vi "Functional Imaging-Update UI element limits.vi"(8 "error in (no error)":errorcluster) -> (0 "error out":errorcluster)   [LabVIEW 2017]
uses:
  Experiment header interface/Typedefs/Header file interface module functions enum.ctl
  Typedefs/Get-Set-Clear Control.ctl
  Global variables/gl_Functional Imaging-Global variables.vi
panel:
  out "Experiment data folder path":path
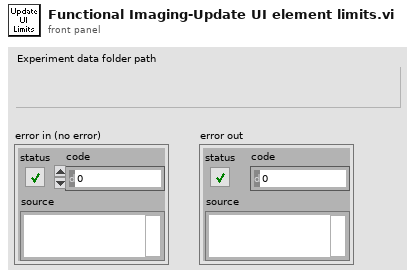
[diagram p1: front panel]
types:
  T1 = typedef "Header file interface module functions enum.ctl" = enum16{"Load experiment header file", "Save experiment header file", "Clear stored values", "Read stored values", "Update specific value in memory", "Update values in memory"}
  T2 = typedef "Functional Imging UI Refs.ctl" = cluster{"Menu ref":refnum<k9>, "Image control":refnum<vi>, "VI ref":refnum<vi>, "XGrapher":refnum<vi>, "Smoothing":refnum<vi>, "POI Averaging":refnum<vi>, "Normalize":refnum<vi>, "POI data points in each trial":refnum<vi>, "Channel":refnum<vi>, "Experiment data folder path":refnum<vi>, "[ROI vis]":refnum<vi>, "[Groups] visbl":T3, "Group Name":refnum<vi>, "POI index":refnum<vi>, "Trial No.":refnum<vi>, "Intensity Zoom":refnum<vi>, "Trial Cursor Enabled":refnum<vi>, "Number of Trials (ind 1)":refnum<vi>, "Number of Trials (ind 2)":refnum<vi>, "MiniScans Available":refnum<vi>, "POI Available":refnum<vi>, "Defer graph updates":refnum<vi>, "Waveform selector":refnum<vi>, "#of selected POI":refnum<vi>, "#of selected MiniScans":refnum<vi>, "#of selected groups":refnum<vi>, "Max Z-Projection":refnum<vi>, "Z-Plane Selector":refnum<vi>, "Index of miniscan point to visualise":refnum<vi>, "ROI vis. mode":refnum<vi>, "Total # of points":refnum<vi>, "Index of group clicked on":refnum<vi>, "Pane 1":refnum<vi>, "Pane 2":refnum<vi>, "Pane 3":refnum<vi>, "Pane 4":refnum<vi>, "Pane 5":refnum<vi>, "Pane 6":refnum<vi>, "Deselect all ROI":refnum<vi>, "Deselect all groups":refnum<vi>}
  T3 = typedef "Groups array referecne.ctl" = refnum<vi>
  T4 = typedef "Header parameters cluster-ALL.ctl" = cluster{"LOGIN":T5, "GLOBAL PARAMETERS":T6, "IMAGING MODES":T8, "TIME SERIES":T9, "MOTOR Z-STACK ":T11, "AOL Z-STACK":T12, "FUNCTIONAL IMAGING":T13, "MOVEMENT CORRECTION":T14, "CALIBRATION":T16, "STATISTICS":T17, "BIOLOGY INFORMATION":T18}
  T5 = typedef "Header params -Login.ctl" = cluster{"User":string, "Profile":string, "Software Version":string, "Experiment Date Time":timestamp}
  T6 = typedef "Header params-Global Parameters.ctl" = cluster{"MicroscopeID":string, "Microscope Type":string, "Objective":string, "Field of View (um)":dbl, "Fill time (us)":dbl, "Experiment Type":T7, "Stimuli Trigger":bool, "Speed Logging":bool}
  T7 = typedef "Experiment Type.ctl" = enum16{"In vivo", "In vitro", "Testing", "Calibration", "Other"}
  T8 = typedef "Header params-Imaging Modes.ctl" = cluster{"Time Series":bool, "Motor Zstack":bool, "AOL Zstack":bool, "Functional Imaging":bool}
  T9 = typedef "Header params-Time Series.ctl" = cluster{"Basic Image meta data":T10, "AOL z":dbl}
  T10 = typedef "Header params-Basic image meta data.ctl" = cluster{"Wavelength (nm)":dbl, "# averaged frames":dbl, "laser power (%)":dbl, "Pockels":dbl, "pixel dwell time (us)":dbl, "fill time (us)":dbl, "pmt 1":dbl, "pmt 2":dbl, "back apperture":dbl, "zoom":dbl, "field of view":dbl, "frame size":dbl, "AOL x centre":dbl, "AOL y centre":dbl, "Stage x position":dbl, "Stage y position":dbl, "Stage z position":dbl}
  T11 = typedef "Header params-Motor Z-stack.ctl" = cluster{"Hdr Basic Image meta data":T10, "Z Start":dbl, "Z Stop":dbl, "No of Planes":dbl}
  T12 = typedef "Header params-AOL Z-stack.ctl" = cluster{"Hdr Basic Image meta data":T10, "Z Start":dbl, "Z Stop":dbl, "No of Planes":dbl}
  T13 = typedef "Header params-Functional Imaging.ctl" = cluster{"Functional Mode":enum16{"Point", "Line", "Patch", "Plane", "Volume"}, "Pockels Modulation":bool, "Number of pois":dbl, "Number of miniscans":dbl, "Number of cycles":dbl, "Number of trials":dbl, "Miniscan dwell time per pixel (us)":dbl, "poi dwell time":dbl, "Rectangle ROI length":dbl, "Rectangle ROI height":dbl, "AOL mode":dbl, "Plane mode":dbl, "video length (sec)":dbl, "Frame rate (fps)":dbl, "Stimuli Timing (usec)":dbl, "Acquisition Length":dbl, "Basic Image meta data":T10, "Z Start (um)":dbl, "Z Stop (um)":dbl}
  T14 = typedef "Header params-Movement correction.ctl" = cluster{"Movement Correction":bool, "Axial Reference":bool, "Reference Size":dbl, "Reference Source":T15, "Reference dwell time (us)":dbl, "Number of Z lines":dbl, "Size of Z pixels":dbl, "Axial Pixels":dbl, "Reference Zoom":dbl, "Reference Average":dbl, "Proportional Scale":dbl, "Integral Scale":dbl, "Proportional Scale Z":dbl, "Integral Scale Z":dbl, "Scan Interval":dbl, "Ref Plot Refresh Rate":dbl}
  T15 = typedef "Reference source.ctl" = enum16{"Green channel", "Red channel"}
  T16 = typedef "Header params-Calibration Setup.ctl" = cluster{"Pockels Calibration File":path, "Calibration_ini file":path, "Setup_ini file":path}
  T17 = typedef "Header params-statistics.ctl" = cluster{"Z-stack duration (sec)":dbl, "Number of acquired data-points":dbl, "Acquisition time (ms)":dbl, "Number of acquired frames":dbl}
  T18 = typedef "Biology Information.ctl" = cluster{"Animal Code or Name":string, "Animal DoB":string, "Animal Age":string, "Animal Sex":string, "Animal Weight":string, "Date of Injection":string, "Date of Implant":string, "Site of Injection":string, "Animal Ear Notch":string, "AAV constructs":string, "Genetic background":string, "Optical reporter":string, "Region of brain imaged":string, "Other \ncomments":string}
  T19 = typedef "Get-Set-Clear Control.ctl" = enum16{"Get", "Set", "Clear"}
  T20 = typedef "Fixed strings.ctl" = cluster{"ROI file name":string, "Normalised ROI file name":string, "Zplane Pockels values file name":string, "Functional data folder name":string, "Experiment Header file name":string, "Z-stack images folder name":string, "Groups setup rel. path":string, "Groups text file rel. path":string, "TDMS files folder name (F.img)":string, "TDMS files folder name (V.acq)":string, "TDMS files folder name (Pl.acq)":string, "Cycle rel times sequence file":string, "Dynamically called VIs folder name":string, "Time Series folder base name":string}
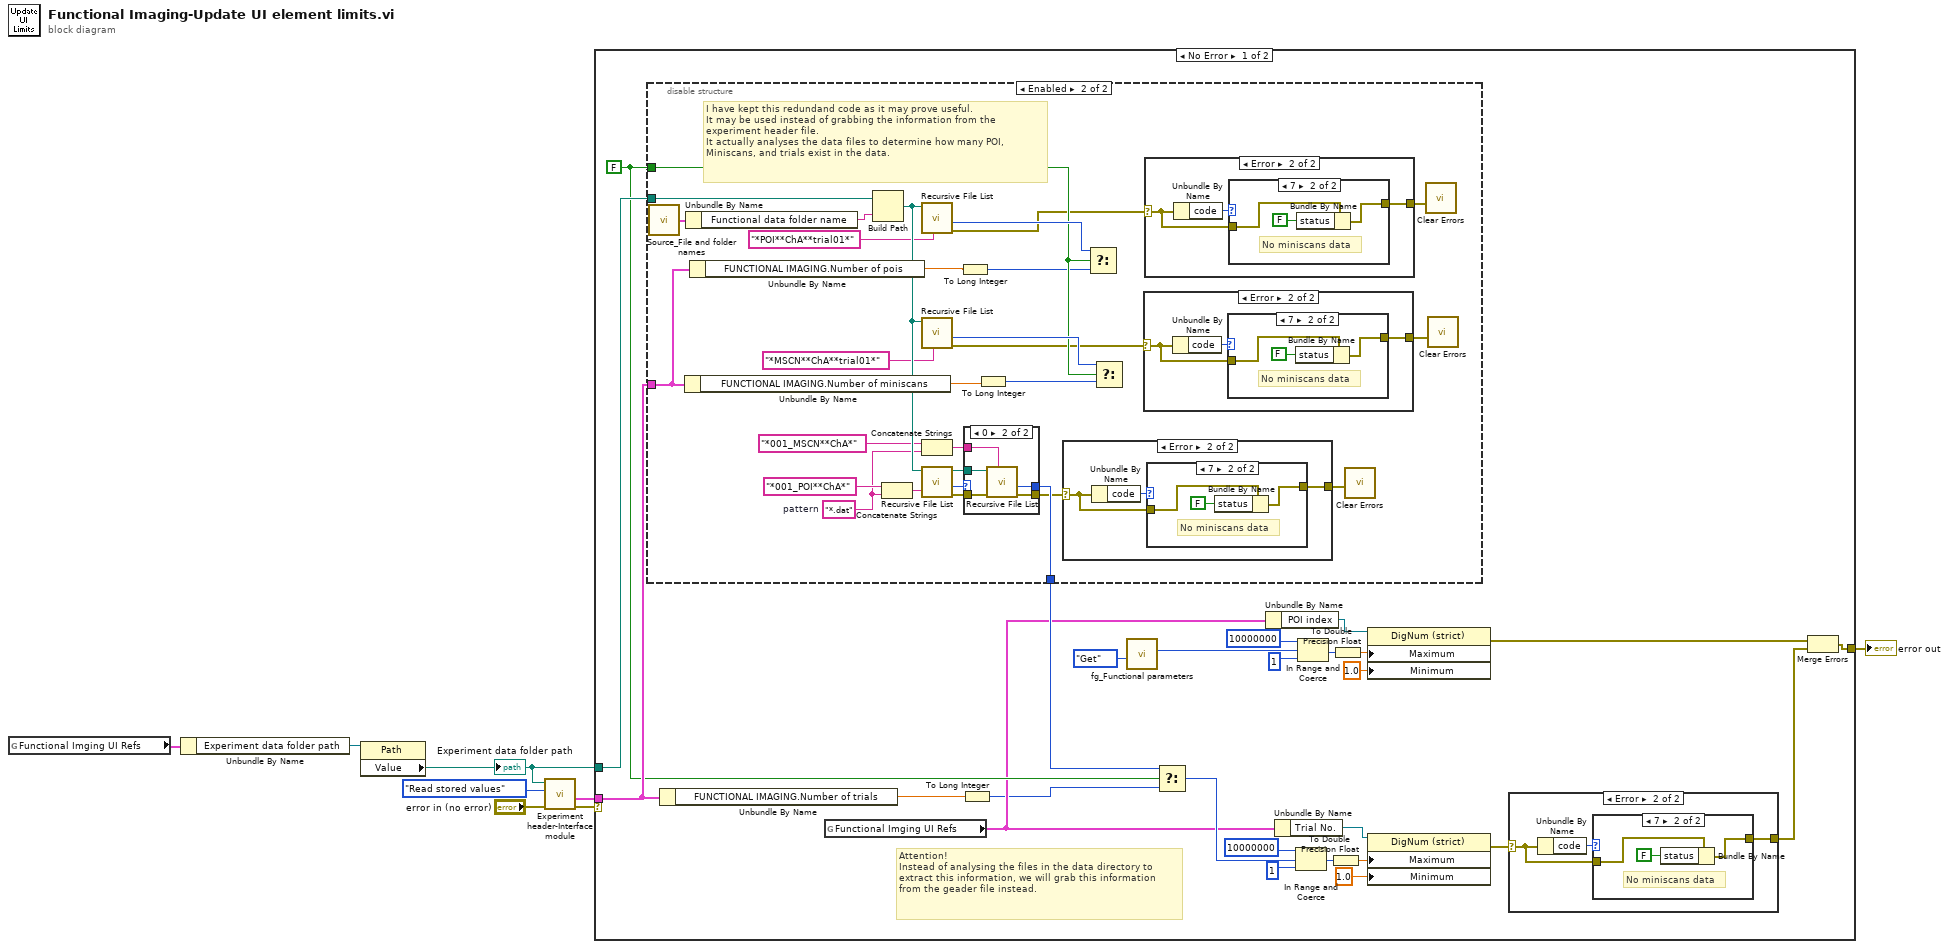
[diagram p0: block diagram]
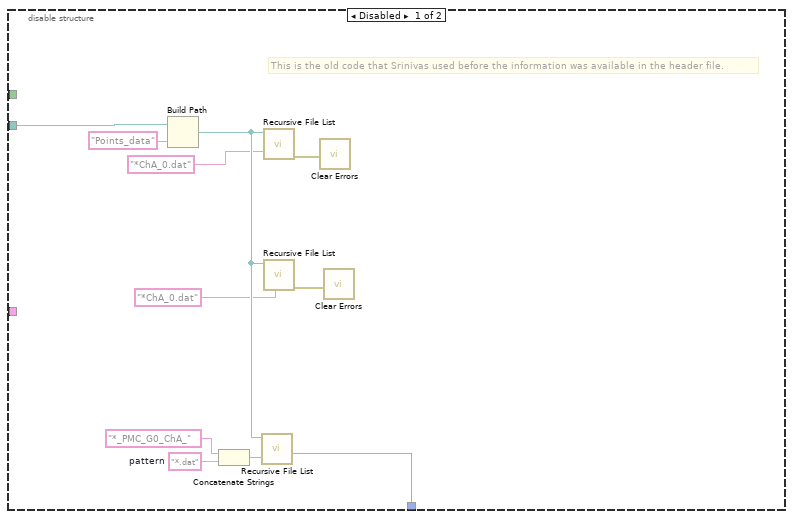
[diagram p2: hidden frame]
diagram:
  n1 = global read "gl_Functional Imaging-Global variables.vi" "Functional Imging UI Refs"() -> (w2:T2)
  n2 = Unbundle By Name(w2) -> ("Experiment data folder path"=w3:refnum<vi>)
  n3 = property class="Path"(reference=w3) -> ("Value"=w1:path)  [unwired: 1 in, 2 out]
  "Experiment data folder path" <- w1
  n4 = call "Experiment header-Interface module.vi"("error in (no error)"="error in (no error)", "Function"=Header_file_interface_module_functions_enum."Read stored values", "Experiment data folder path"=w1) -> ("error out"=w4:errorcluster, "All header parameters out"=w7:T4)  [unwired: 7 in]
  n5 = case shown="No Error" w4 {
    selector: w4 -> [_ w114]
    tunnel: w1 -> [w30 _]
    tunnel: [w31 w114] -> w8
    tunnel: w7 -> [w18 _]
    frame No Error {
      w13 = FALSE ("s")
      # "Attention!\nInstead of analysing the files in the data directory to extract this information, we will grab this information from the geader file instead."
      n6 = disable-structure shown="Enabled" {
        disable-tunnel: w30 -> [w45 w74]
        disable-tunnel: w18 -> [_ w73]
        disable-tunnel: [w41 w70] -> w14
        disable-tunnel: w13 -> [_ w59]
        frame Disabled {
          w37 = "*.dat"  # pattern
          # "This is the old code that Srinivas used before the information was available in the header file."
          n7 = Build Path(base path=w45, name or relative path="Points_data") -> (appended path=w40:path)
          n8 = Concatenate Strings("*_PMC_G0_ChA_" ("string"), w37) -> (w38:string)
          n9 = call <vilib>:"Recursive File List.vi"("pattern"=w38, "Folder Path"=w40) -> ("Number of Files"=w41:i32)  [unwired: 5 in, 4 out]
          n10 = call <vilib>:"Recursive File List.vi"("pattern"="*ChA_0.dat", "Folder Path"=w40) -> ("error out"=w43:errorcluster)  [unwired: 5 in, 4 out]
          n11 = call <vilib>:"Recursive File List.vi"("pattern"="*ChA_0.dat", "Folder Path"=w40) -> ("error out"=w42:errorcluster)  [unwired: 5 in, 4 out]
          n12 = call <vilib>:"Clear Errors.vi"("error in (no error)"=w43) -> ()  [unwired: 5 in, 2 out]
          n13 = call <vilib>:"Clear Errors.vi"("error in (no error)"=w42) -> ()  [unwired: 5 in, 2 out]
        }
        frame Enabled {
          w52 = "*.dat"  # pattern
          # "I have kept this redundand code as it may prove useful.\nIt may be used instead of grabbing the information from the experiment header file.\nIt actually analyses the data files to determine how many POI, Miniscans, and trials exist in the data."
          n14 = call "Source_File and folder names.vi"() -> ("Fixed strings"=w50:T20)  [unwired: 1 in]
          n15 = Unbundle By Name(w73) -> ("FUNCTIONAL IMAGING.Number of miniscans"=w47:dbl)
          n16 = Unbundle By Name(w50) -> ("Functional data folder name"=w51:string)
          n17 = Unbundle By Name(w73) -> ("FUNCTIONAL IMAGING.Number of pois"=w49:dbl)
          n18 = Build Path(base path=w74, name or relative path=w51) -> (appended path=w69:path)
          n19 = Concatenate Strings("*001_POI**ChA*" ("string"), w52) -> (w65:string)
          n20 = call <vilib>:"Recursive File List.vi"("pattern"="*POI**ChA**trial01*", "Folder Path"=w69) -> ("error out"=w56:errorcluster, "Number of Files"=w72:i32)  [unwired: 5 in, 3 out]
          n21 = call <vilib>:"Recursive File List.vi"("pattern"="*MSCN**ChA**trial01*", "Folder Path"=w69) -> ("error out"=w57:errorcluster, "Number of Files"=w71:i32)  [unwired: 5 in, 3 out]
          n22 = Concatenate Strings("*001_MSCN**ChA*" ("string"), w52) -> (w61:string)
          n23 = call <vilib>:"Recursive File List.vi"("pattern"=w65, "Folder Path"=w69) -> ("error out"=w64:errorcluster, "Number of Files"=w63:i32, "dup Folder Path"=w60:path)  [unwired: 5 in, 2 out]
          n24 = To Long Integer(number=w49) -> (32bit integer=w48:i32)
          n25 = case shown="0" w63 {
            selector: w63 -> [w100 _]
            tunnel: w64 -> [w99 w104]
            tunnel: [w100 w103] -> w70
            tunnel: [w99 w105] -> w58
            tunnel: w61 -> [_ w102]
            tunnel: w60 -> [_ w101]
            frame Default {
            }
            frame 0 {
              n26 = call <vilib>:"Recursive File List.vi"("pattern"=w102, "error in (no error)"=w104, "Folder Path"=w101) -> ("error out"=w105:errorcluster, "Number of Files"=w103:i32)  [unwired: 4 in, 3 out]
            }
          }
          n27 = To Long Integer(number=w47) -> (32bit integer=w46:i32)
          n28 = case shown="Error" w58 {
            selector: w58 -> [w91 w93]
            tunnel: [w91 w92] -> w55
            frame No Error {
            }
            frame Error {
              n29 = Unbundle By Name(w93) -> ("code"=w94:i32)
              n30 = case shown="7" w94 {
                tunnel: w93 -> [w95 w98]
                tunnel: [w95 w96] -> w92
                frame Default {
                }
                frame 7 {
                  # "No miniscans data"
                  n31 = Bundle By Name(cluster=w98, "status"=FALSE) -> (w96:errorcluster)
                }
              }
            }
          }
          n32 = Select(t=w72, s=w59, f=w48) -> ()  [unwired: 1 out]
          n33 = Select(t=w71, s=w59, f=w46) -> ()  [unwired: 1 out]
          n34 = case shown="Error" w57 {
            selector: w57 -> [w83 w85]
            tunnel: [w83 w84] -> w53
            frame No Error {
            }
            frame Error {
              n35 = Unbundle By Name(w85) -> ("code"=w86:i32)
              n36 = case shown="7" w86 {
                tunnel: w85 -> [w87 w90]
                tunnel: [w87 w88] -> w84
                frame Default {
                }
                frame 7 {
                  # "No miniscans data"
                  n37 = Bundle By Name(cluster=w90, "status"=FALSE) -> (w88:errorcluster)
                }
              }
            }
          }
          n38 = case shown="Error" w56 {
            selector: w56 -> [w75 w77]
            tunnel: [w75 w76] -> w54
            frame No Error {
            }
            frame Error {
              n39 = Unbundle By Name(w77) -> ("code"=w78:i32)
              n40 = case shown="7" w78 {
                tunnel: w77 -> [w79 w82]
                tunnel: [w79 w80] -> w76
                frame Default {
                }
                frame 7 {
                  # "No miniscans data"
                  n41 = Bundle By Name(cluster=w82, "status"=FALSE) -> (w80:errorcluster)
                }
              }
            }
          }
          n42 = call <vilib>:"Clear Errors.vi"("error in (no error)"=w55) -> ()  [unwired: 5 in, 2 out]
          n43 = call <vilib>:"Clear Errors.vi"("error in (no error)"=w54) -> ()  [unwired: 5 in, 2 out]
          n44 = call <vilib>:"Clear Errors.vi"("error in (no error)"=w53) -> ()  [unwired: 5 in, 2 out]
        }
      }
      n45 = Unbundle By Name(w18) -> ("FUNCTIONAL IMAGING.Number of trials"=w10:dbl)
      n46 = global read "gl_Functional Imaging-Global variables.vi" "Functional Imging UI Refs"() -> (w11:T2)
      n47 = To Long Integer(number=w10) -> (32bit integer=w9:i32)
      n48 = call "fg_Functional parameters.vi"("Function"=Get-Set-Clear_Control."Get") -> ("# of ROI"=w16:i32)  [unwired: 7 in, 3 out]
      n49 = Select(t=w14, s=w13, f=w9) -> (s? t:f=w15:i32)
      n50 = Unbundle By Name(w11) -> ("POI index"=w32:refnum<vi>)
      n51 = Unbundle By Name(w11) -> ("Trial No."=w21:refnum<vi>)
      n52 = In Range and Coerce(upper limit=10000000, x=w15, lower limit=1) -> (coerced(x)=w25:i32)  [unwired: 1 out]
      n53 = In Range and Coerce(upper limit=10000000, x=w16, lower limit=1) -> (coerced(x)=w27:i32)  [unwired: 1 out]
      n54 = To Double Precision Float(number=w25) -> (double precision float=w22:dbl)
      n55 = To Double Precision Float(number=w27) -> (double precision float=w26:dbl)
      n56 = property on="Property Node" class="DigNum (strict)"(reference=w32, "Maximum"=w26, "Minimum"=1.0 ("Data Entry Limits:Minimum")) -> (error out=w12:errorcluster)  [unwired: 1 in, 1 out]
      n57 = property on="Property Node" class="DigNum (strict)"(reference=w21, "Maximum"=w22, "Minimum"=1.0 ("Data Entry Limits:Minimum")) -> (error out=w20:errorcluster)  [unwired: 1 in, 1 out]
      n58 = case shown="Error" w20 {
        selector: w20 -> [w106 w108]
        tunnel: [w106 w107] -> w19
        frame No Error {
        }
        frame Error {
          n59 = Unbundle By Name(w108) -> ("code"=w109:i32)
          n60 = case shown="7" w109 {
            tunnel: w108 -> [w110 w113]
            tunnel: [w110 w111] -> w107
            frame Default {
            }
            frame 7 {
              # "No miniscans data"
              n61 = Bundle By Name(cluster=w113, "status"=FALSE) -> (w111:errorcluster)
            }
          }
        }
      }
      n62 = Merge Errors(w12, w19) -> (w31:errorcluster)
    }
    frame Error {
    }
  }
  "error out" <- w8
